vi "Reset Sensors.vi"   [LabVIEW 2014]
uses:
  Common Code/Elevator Mode.ctl
  Elevator/Elevator Command.ctl
  Elevator/Elevator Control Command.ctl
  Common Code/Elevator Idle Mode.ctl
  Robot Global Data.vi
types:
  T1 = typedef "Elevator Idle Mode.ctl" = enum16{"Load 1", "Load 2", "Load 3", "Load Can", "Untip Can", "Step Load", "Drop Stack"}
  T2 = typedef "Elevator Control Command.ctl" = cluster{"Command":T3, "Manual Motor Out":dbl, "Manual Eject Piston":bool, "Mode":T4, "Override Limits":bool, "Manual Stabilizer":bool, "Manual Finger":bool, "Store Trashcan?":bool, "Hold Low?":bool, "Idle Mode":T1, "HP Load":bool, "Unstick":bool}
  T3 = typedef "Elevator Command.ctl" = enum16{"Idle", "Load 1", "Load 2", "Load 3", "Drop Stack", "Eject Stack", "Untip Trashcan", "Load Trashcan", "HP Load", "HP Score"}
  T4 = typedef "Elevator Mode.ctl" = enum16{"Manual", "Safe", "Auto"}
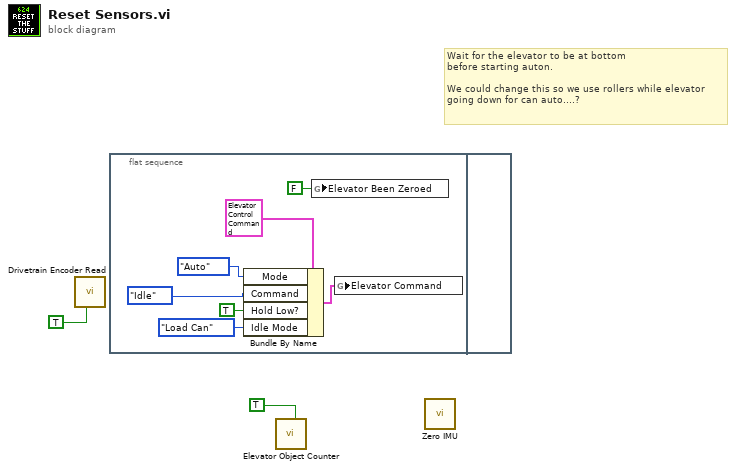
[diagram p0: block diagram]
diagram:
  # "Wait for the elevator to be at bottom\nbefore starting auton.\n\nWe could change this so we use rollers while elevator\ngoing down for can auto....?"
  n1 = call "Drivetrain Encoder Read.vi"("Reset?"=TRUE) -> ()  [unwired: 10 in, 1 out]
  n2 = flat-sequence {
    frame #0 {
      n3 = Bundle By Name(cluster=T2 {"Command"=enum."Idle", "Manual Motor Out"=0.0, "Manual Eject Piston"=FALSE, "Mode"=enum."Manual", "Override Limits"=FALSE, "Manual Stabilizer"=FALSE, "Manual Finger"=FALSE, "Store Trashcan?"=FALSE, "Hold Low?"=FALSE, "Idle Mode"=enum."Load 1", "HP Load"=FALSE, "Unstick"=FALSE} ("Elevator Command"), "Mode"=Elevator_Mode."Auto", "Command"=Elevator_Command."Idle", "Hold Low?"=TRUE, "Idle Mode"=Elevator_Idle_Mode."Load Can") -> (w7:T2)
      n4 = global write "Robot Global Data.vi" "Elevator Been Zeroed"(FALSE ("Elevator Been Zeroed")) -> ()
      n5 = global write "Robot Global Data.vi" "Elevator Command"(w7) -> ()
    }
    frame #1 {
    }
  }
  n6 = call "Elevator Object Counter.vi"("Clear Stack?"=TRUE) -> ()  [unwired: 9 in, 2 out]
  n7 = call "Zero IMU.vi"() -> ()  [unwired: 12 in]
